vi "Str Convert COM.vi"(5 "COM":string="COM15,9600,8,0,10,0") -> (2 "COM Out":T1={"VISA"="", "baud rate"=9600, "data bits"=8, "parity"=enum."None", "stop bits"=10, "flow control"=0} {"flow control" items=["None", "XON/XOFF", "RTS/CTS", "XON/XOFF & RTS/CTS", "DTR/DSR", "XON/XOFF & DTR/DSR"]; "stop bits" items=["1.0"=10, "1.5"=15, "2.0"=20]})   [LabVIEW 2014]
uses:
  Ctr/VISA Ctr.ctl
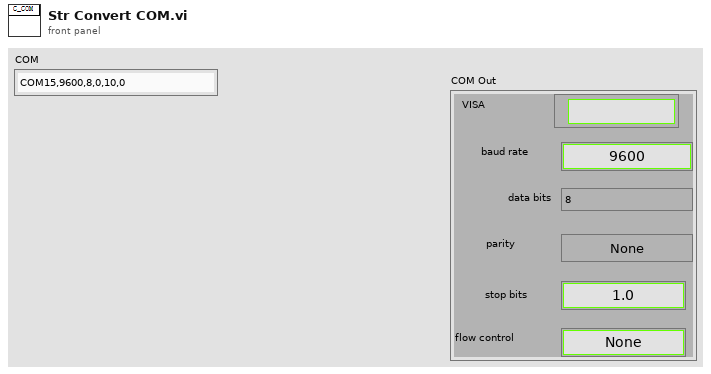
[diagram p1: front panel]
types:
  T1 = typedef "VISA Ctr.ctl" = cluster{"VISA":refnum<visa-resource-name>, "baud rate":u32, "data bits":u16, "parity":enum16{"None", "Odd", "Even", "Mark", "Space"}, "stop bits":u16, "flow control":u16}
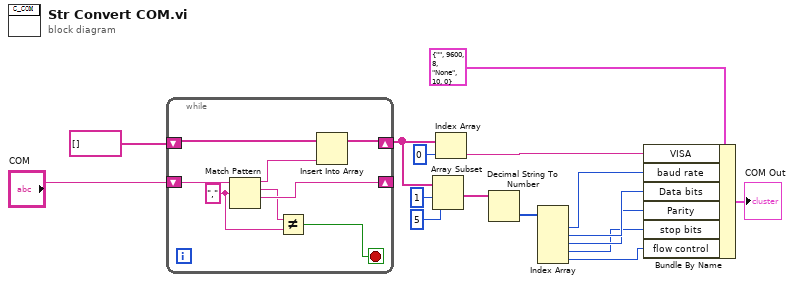
[diagram p0: block diagram]
diagram:
  n1 = while {
    shift-right: [w17] -> w11
    shift-left: string[] [] -> [w23]
    shift-right: [w21] -> _
    shift-left: "COM" -> [w24]
    stop <- w18 stop-if-true
    w19 = "," ("正则表达式")
    n2 = Match Pattern(string=w24, regular expression=w19) -> (before substring=w22:string, match substring=w20:string, after substring=w21:string)  [unwired: 1 in, 1 out]
    n3 = Not Equal?(x=w20, y=w19) -> (x != y?=w18:bool)
    n4 = Insert Into Array(array=w23, new element=w22) -> (w17:string[])  [unwired: 1 in]
  }
  n5 = Array Subset(array=w11, index=1 ("索引"), length=5 ("长度")) -> (w8:string[])
  n6 = Index Array(array=w11, index=0 ("索引")) -> (element=w12:string)
  n7 = Decimal String To Number(string=w8) -> (number=w7:i32[])  [unwired: 2 in, 1 out]
  n8 = Index Array(array=w7) -> (element #1=w6:i32, element #2=w5:i32, element #3=w4:i32, element #4=w3:i32, element #5=w2:i32)  [unwired: 5 in]
  n9 = Bundle By Name(cluster=T1 {"VISA"="", "baud rate"=9600, "data bits"=8, "parity"=enum."None", "stop bits"=10, "flow control"=0} ("VISA"), "VISA"=w12, "baud rate"=w6, "Data bits"=w5, "Parity"=w4, "stop bits"=w3, "flow control"=w2) -> (→"COM Out":T1)
